vi "DelayLineInit.vi"(1 "Inst bool":u64, 2 "Inst_param":T1) -> ()   [LabVIEW 2013]
uses:
  Drivers/Set Parameter.ctl
  Drivers/Get Parameter.ctl
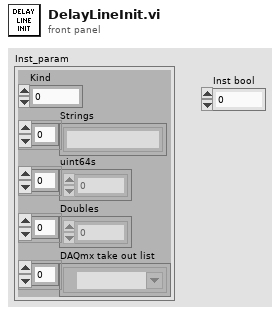
[diagram p1: front panel]
types:
  T1 = cluster{"Kind":u16, "Strings":string[], "uint64s":u64[], "Doubles":dbl[], "DAQmx take out list":refnum<k21>[]}
  T2 = typedef "Set Parameter.ctl" = enum16{"Acceleration (A)", "Baud Rate (BD)", "Counter 1 (C1)", "Counter 2 (C2)", "Control C Software Reset (CE)", "Check Sum Enable (CK)", "Clock Mode (CM)", "Clock Mode Ratio (CR)", "Clock Mode Out Step Width (CW)", "Deceleration (D)", "Digital Filtering, Input 1 (D1)", "Digital Filtering, Input 2 (D2)", "Digital Filtering, Input 3 (D3)", "Digital Filtering, Input 4 (D4)", "Digital Filtering, Input 5 (D5)", "Digital Filtering, Input 9 (D9)", "Digital Filtering, Input 10 (D10)", "Digital Filtering, Input 11 (D11)", "Digital Filtering, Input 12 (D12)", "Deadband (DB)", "Decrement Variable (DC)", "Enable/Disable Drive (DE)", "Device Name (DN)", "End Program Execution (E)", "Encoder Function Enable (EE)", "Encoder Lines (EL)", "Echo Mode (EM)", "Escape (ES)", "Execute Program at Address (EX)", "Hold (H)", "Hold Current (HC)", "Hold Current Delay Time (HI)", "Home to Encoder Index (HM)", "Home to Home Switch (HT)", "Increment Variable (IC)", "Initialize Parameters to NVM (IP)", "Input into Variable (IV)", "Jog Enable (JE)", "Limit Stop Mode (LM)", "Move Absolute (MA)", "Move Relative (MR)", "MicroStepping Select (MS)", "Motor Settling Delay Time (MT)", "Output 1 (O1)", "Output 2 (O2)", "Output 3 (O3)", "Output 4 (O4)", "Output 9 (O9)", "Output 10 (O10)", "Output 11 (O11)", "Output 12 (O12)", "Output High Byte (9-12) (OH)", "Output Low Byte (1-4) (OL)", "Output Total (1-4 and 9-12) (OT)", "Position Maintenance (PM)", "Party Mode (PY)", "Register 1 (R1)", "Register 2 (R2)", "Register 3 (R3)", "Register 4 (R4)", "Run Current (RC)", "Stall Factor (SF)", "Slew (SL)", "Stall Mode Set (SM)", "Upgrade Firmware (UG)", "Velocity Initial (VI)", "Velocity Maximum (VM)"}
  T3 = typedef "Get Parameter.ctl" = enum16{"Acceleration (A)", "Baud Rate (BD)", "Busy Flag (BY)", "Counter 1 (C1)", "Counter 2 (C2)", "Check Sum Enable (CK)", "Clock Mode (CM)", "Clock Mode Ratio (CR)", "Clock Mode Out Step Width (CW)", "Deceleration (D)", "Digital Filtering, Input 1 (D1)", "Digital Filtering, Input 2 (D2)", "Digital Filtering, Input 3 (D3)", "Digital Filtering, Input 4 (D4)", "Digital Filtering, Input 5 (D5)", "Digital Filtering, Input 9 (D9)", "Digital Filtering, Input 10 (D10)", "Digital Filtering, Input 11 (D11)", "Digital Filtering, Input 12 (D12)", "Deadband (DB)", "Enable/Disable Drive (DE)", "Device Name (DN)", "End Program Execution (E)", "Encoder Function Enable (EE)", "Encoder Lines (EL)", "Error Flag (EF)", "Error Variable (ER)", "Echo Mode (EM)", "Escape (ES)", "Execute Program at Address (EX)", "Hold Current (HC)", "Hold Current Delay Time (HI)", "Input 1 (I1)", "Input 2 (I2)", "Input 3 (I3)", "Input 4 (I4)", "Input 5 Analog (I5)", "Input 6 Encoder Index (I6)", "Input 9 (I9)", "Input 10 (I10)", "Input 11 (I11)", "Input 12 (I12)", "Input Low Byte (1-4) (IL)", "Input High Byte (9-12) (IH)", "Inputs Total (1-4,9-12) (IN)", "Internal Temperature (IT)", "Jog Enable (JE)", "Limit Stop Mode (LM)", "MicroStepping Select (MS)", "Motor Settling Delay Time (MT)", "Moving Flag (MV)", "Output 1 (O1)", "Output 2 (O2)", "Output 3 (O3)", "Output 4 (O4)", "Output 9 (O9)", "Output 10 (O10)", "Output 11 (O11)", "Output 12 (O12)", "Output High Byte (9-12) (OH)", "Output Low Byte (1-4) (OL)", "Output Total (1-4 and 9-12) (OT)", "Position Captured at Trip (PC)", "Position Maintenance (PM)", "Part Number (PN)", "Party Mode (PY)", "Register 1 (R1)", "Register 2 (R2)", "Register 3 (R3)", "Register 4 (R4)", "Run Current (RC)", "Serial Number (SN)", "Stall Flag (ST)", "Stall Factor (SF)", "Stall Mode Set (SM)", "User Variables (UV)", "Velocity (V)", "Velocity Changing Flag (VC)", "Velocity Initial (VI)", "Version, Firmware (VR)", "Velocity Maximum (VM)"}
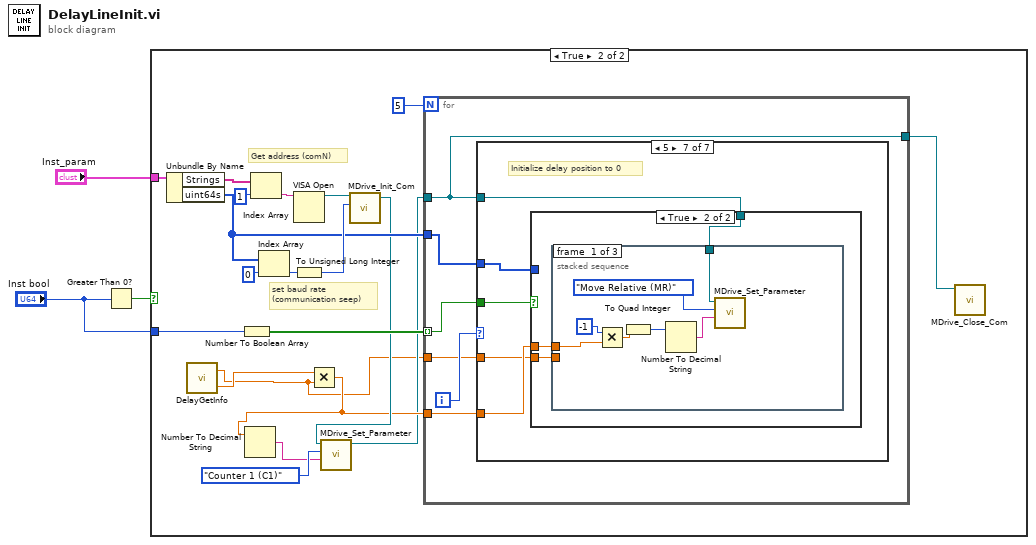
[diagram p0: block diagram]
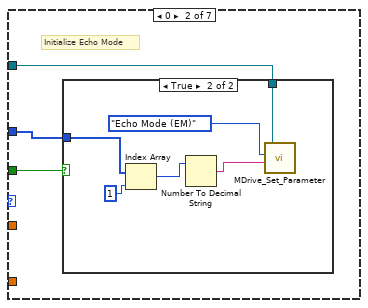
[diagram p4: hidden frame]
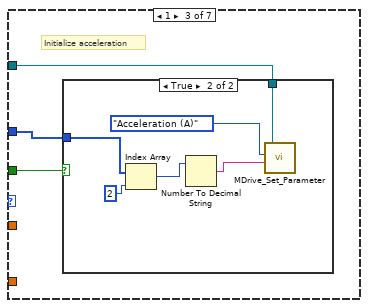
[diagram p6: hidden frame]
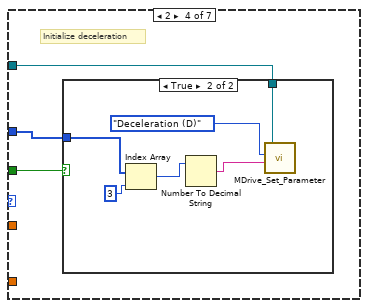
[diagram p8: hidden frame]
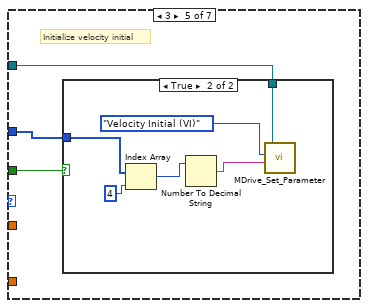
[diagram p10: hidden frame]
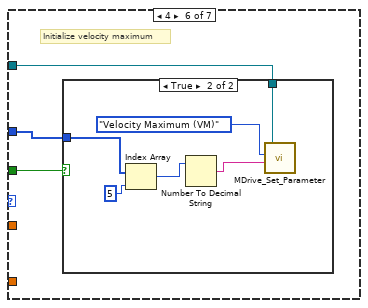
[diagram p12: hidden frame]
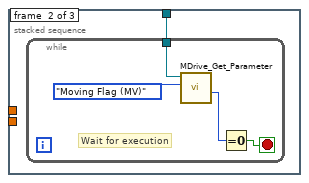
[diagram p15: hidden frame]
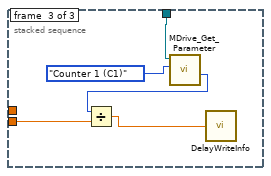
[diagram p16: hidden frame]
diagram:
  n1 = Greater Than 0?(x="Inst bool") -> (x > 0?=w3:bool)
  n2 = case shown="True" w3 {
    tunnel: "Inst_param" -> [_ w23]
    tunnel: "Inst bool" -> [_ w15]
    frame False {
    }
    frame True {
      # "Get address (comN)"
      # "set baud rate\n(communication seep)"
      n3 = Unbundle By Name(w23) -> ("Strings"=w22:string[], "uint64s"=w12:u64[])
      n4 = call "DelayGetInfo.vi"() -> ("Delay position (ps)"=w5:dbl, "Conversion"=w4:dbl)  [unwired: 2 in]
      n5 = Number To Boolean Array(number=w15) -> (Boolean array=w14:bool[])
      n6 = Index Array(array=w22, index=1) -> (element=w20:string)
      n7 = Index Array(array=w12, index=0) -> (element=w17:u64)
      n8 = VISA Open(VISA resource name=w20) -> (VISA resource name=w19:refnum<visa-resource-name>)  [unwired: 4 in, 1 out]
      n9 = To Unsigned Long Integer(number=w17) -> (unsigned 32bit integer=w16:u32)
      n10 = Multiply(x=w5, y=w4) -> (x*y=w7:dbl)
      n11 = Number To Decimal String(number=w7) -> (decimal integer string=w9:string)  [unwired: 1 in]
      n12 = call "MDrive_Init_Com.vi"("VISA resource name"=w19, "baud rate"=w16) -> ("VISA resource name out"=w8:refnum<visa-resource-name>)  [unwired: 5 in, 1 out]
      n13 = call "MDrive_Set_Parameter.vi"("Parameter Setpoint"=w9, "Set Parameter"=Set_Parameter."Counter 1 (C1)", "VISA resource name out 2"=w8) -> ("VISA resource name out"=w6:refnum<visa-resource-name>)  [unwired: 2 in, 2 out]
      n14 = for {
        N: 5 -> [_]
        tunnel: w14 -> [w27] mode=indexing
        tunnel: w12 -> [w29]
        tunnel: w6 -> [w26]
        tunnel: [w26] -> w11
        tunnel: w7 -> [w25]
        tunnel: w4 -> [w24]
        i -> [w28]
        n15 = case shown="5" w28 {
          tunnel: w29 -> [_ w31 w40 w49 w58 w67 w78]
          tunnel: w27 -> [_ w32 w41 w50 w59 w68 w79]
          tunnel: w26 -> [_ w30 w39 w48 w57 w66 w77]
          tunnel: w25 -> [_ _ _ _ _ _ w76]
          tunnel: w24 -> [_ _ _ _ _ _ w75]
          frame 100, Default {
          }
          frame 0 {
            # "Initialize Echo Mode"
            n16 = case shown="True" w32 {
              tunnel: w31 -> [_ w34]
              tunnel: w30 -> [_ w33]
              frame False {
              }
              frame True {
                n17 = Index Array(array=w34, index=1) -> (element=w36:u64)
                n18 = Number To Decimal String(number=w36) -> (decimal integer string=w35:string)  [unwired: 1 in]
                n19 = call "MDrive_Set_Parameter.vi"("Parameter Setpoint"=w35, "Set Parameter"=Set_Parameter."Echo Mode (EM)", "VISA resource name out 2"=w33) -> ()  [unwired: 2 in, 3 out]
              }
            }
          }
          frame 1 {
            # "Initialize acceleration"
            n20 = case shown="True" w41 {
              tunnel: w40 -> [_ w43]
              tunnel: w39 -> [_ w42]
              frame False {
              }
              frame True {
                n21 = Index Array(array=w43, index=2) -> (element=w45:u64)
                n22 = Number To Decimal String(number=w45) -> (decimal integer string=w44:string)  [unwired: 1 in]
                n23 = call "MDrive_Set_Parameter.vi"("Parameter Setpoint"=w44, "Set Parameter"=Set_Parameter."Acceleration (A)", "VISA resource name out 2"=w42) -> ()  [unwired: 2 in, 3 out]
              }
            }
          }
          frame 2 {
            # "Initialize deceleration"
            n24 = case shown="True" w50 {
              tunnel: w49 -> [_ w52]
              tunnel: w48 -> [_ w51]
              frame False {
              }
              frame True {
                n25 = Index Array(array=w52, index=3) -> (element=w54:u64)
                n26 = Number To Decimal String(number=w54) -> (decimal integer string=w53:string)  [unwired: 1 in]
                n27 = call "MDrive_Set_Parameter.vi"("Parameter Setpoint"=w53, "Set Parameter"=Set_Parameter."Deceleration (D)", "VISA resource name out 2"=w51) -> ()  [unwired: 2 in, 3 out]
              }
            }
          }
          frame 3 {
            # "Initialize velocity initial"
            n28 = case shown="True" w59 {
              tunnel: w58 -> [_ w61]
              tunnel: w57 -> [_ w60]
              frame False {
              }
              frame True {
                n29 = Index Array(array=w61, index=4) -> (element=w63:u64)
                n30 = Number To Decimal String(number=w63) -> (decimal integer string=w62:string)  [unwired: 1 in]
                n31 = call "MDrive_Set_Parameter.vi"("Parameter Setpoint"=w62, "Set Parameter"=Set_Parameter."Velocity Initial (VI)", "VISA resource name out 2"=w60) -> ()  [unwired: 2 in, 3 out]
              }
            }
          }
          frame 4 {
            # "Initialize velocity maximum"
            n32 = case shown="True" w68 {
              tunnel: w67 -> [_ w70]
              tunnel: w66 -> [_ w69]
              frame False {
              }
              frame True {
                n33 = Index Array(array=w70, index=5) -> (element=w72:u64)
                n34 = Number To Decimal String(number=w72) -> (decimal integer string=w71:string)  [unwired: 1 in]
                n35 = call "MDrive_Set_Parameter.vi"("Parameter Setpoint"=w71, "Set Parameter"=Set_Parameter."Velocity Maximum (VM)", "VISA resource name out 2"=w69) -> ()  [unwired: 2 in, 3 out]
              }
            }
          }
          frame 5 {
            # "Initialize delay position to 0"
            n36 = case shown="True" w79 {
              tunnel: w78 -> [_ _]
              tunnel: w77 -> [_ w82]
              tunnel: w76 -> [_ w81]
              tunnel: w75 -> [_ w80]
              frame False {
              }
              frame True {
                n37 = stacked-sequence {
                  tunnel: w82 -> [w88 w90 w99]
                  tunnel: w81 -> [w87 _ _]
                  tunnel: w80 -> [_ _ w96]
                  frame #0 {
                    n38 = Multiply(x=-1, y=w87) -> (x*y=w85:dbl)
                    n39 = To Quad Integer(1:w85) -> (0:w83:i64)
                    n40 = Number To Decimal String(number=w83) -> (decimal integer string=w84:string)  [unwired: 1 in]
                    n41 = call "MDrive_Set_Parameter.vi"("Parameter Setpoint"=w84, "Set Parameter"=Set_Parameter."Move Relative (MR)", "VISA resource name out 2"=w88) -> ()  [unwired: 2 in, 3 out]
                  }
                  frame #1 {
                    n42 = while {
                      tunnel: w90 -> [w93]
                      stop <- w91 stop-if-true
                      # "Wait for execution"
                      n43 = call "MDrive_Get_Parameter.vi"("Get Parameter"=Get_Parameter."Moving Flag (MV)", "VISA resource name in"=w93) -> ("Parameter Data Numeric"=w92:i32)  [unwired: 2 in, 3 out]
                      n44 = Equal To 0?(x=w92) -> (x = 0?=w91:bool)
                    }
                  }
                  frame #2 {
                    n45 = call "MDrive_Get_Parameter.vi"("Get Parameter"=Get_Parameter."Counter 1 (C1)", "VISA resource name in"=w99) -> ("Parameter Data Numeric"=w97:i32)  [unwired: 2 in, 3 out]
                    n46 = Divide(x=w97, y=w96) -> (x/y=w95:dbl)
                    n47 = call "DelayWriteInfo.vi"("Delay position input (ps)"=w95) -> ()
                  }
                }
              }
            }
          }
        }
      }
      n48 = call "MDrive_Close_Com.vi"("VISA resource name out"=w11) -> ()  [unwired: 3 in]
    }
  }
